vi "Stop Core.vi"(10 "final error code":i32, 11 "AE75TX in":refnum<class "AE75TX.lvclass">) -> (3 "AE75TX out":refnum<class "AE75TX.lvclass">)   [LabVIEW 2015, in "AE75TX Actor.lvlib" / "AE75TX.lvclass"]
doc: "(<B>Filename</B>: Actor Framework.lvlib:Actor.lvclass:Stop Core.vi)\n\nDefines what the actor does before it stops. Use the <B>final error code</B> input to determine whether the actor shut down in response to an error.\n\nBy default, this method does nothing. A descendant class may override it to define behavior, such as shutting down any processes the actor initiated in its override of the Actor Core method."
uses:
  AE75TX.lvclass
  AE75TX.lvclass/AE75TX.ctl
  <vilib>/ActorFramework/Actor/Actor.lvclass
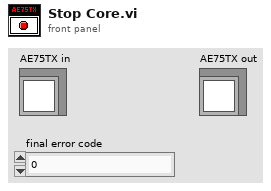
[diagram p1: front panel]
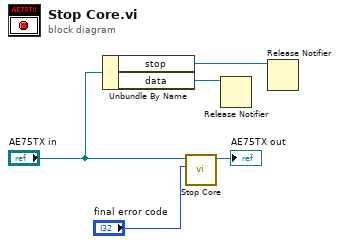
[diagram p0: block diagram]
diagram:
  n1 = Unbundle By Name("AE75TX in") -> ("stop"=w1:refnum<notifier>, "data"=w2:refnum<notifier>)
  n2 = call-parent "Stop Core.vi"("final error code"="final error code", "Actor in"="AE75TX in") -> ("Actor out"=→"AE75TX out":refnum<class "AE75TX.lvclass">)  [unwired: 9 in]
  n3 = Release Notifier(notifier=w2) -> ()  [unwired: 2 in, 3 out]
  n4 = Release Notifier(notifier=w1) -> ()  [unwired: 2 in, 3 out]
